vi "Compare Images DCT.vi"(10 "Image 2":path=path "C:/Users/Matthew/Clients/Users Group/Coding Challenge/Submissions/drt_altered.bmp", 11 "Image 1":path=path "C:/Users/Matthew/Clients/Users Group/Coding Challenge/Submissions/drt.bmp") -> (3 "Hamming Distance":i32)   [LabVIEW 2014, in "Perceptual Hash Comparison.lvclass"]
uses:
  Perceptual Hash Comparison.lvclass
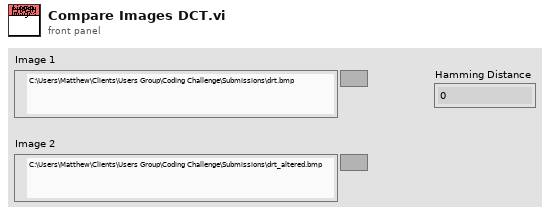
[diagram p1: front panel]
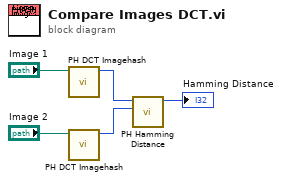
[diagram p0: block diagram]
diagram:
  n1 = call "PH DCT Imagehash.vi"("Image Path"="Image 1") -> ("DCT phash"=w3:u64)  [unwired: 10 in]
  n2 = call "PH DCT Imagehash.vi"("Image Path"="Image 2") -> ("DCT phash"=w2:u64)  [unwired: 10 in]
  n3 = call "PH Hamming Distance.vi"("Hash B"=w2, "Hash A"=w3) -> ("Hamming Distance"=→"Hamming Distance":i32)  [unwired: 9 in]
